vi "Translate XBox Controller Data 2.vi"(2 "Steer Axis":i32, 3 "Drive Axis":dbl) -> (0 "Steer Value Output String":string, 1 "Drive Value Output String":string)   [LabVIEW 2011]
uses:
  <vilib>/express/express arith-compare/Formula/XNode/ExpressFormulaBlockNode.xnode
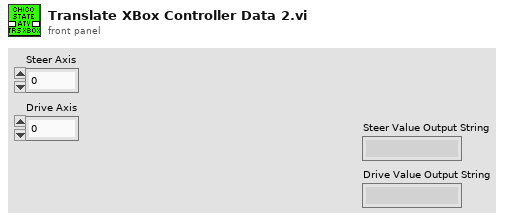
[diagram p1: front panel]
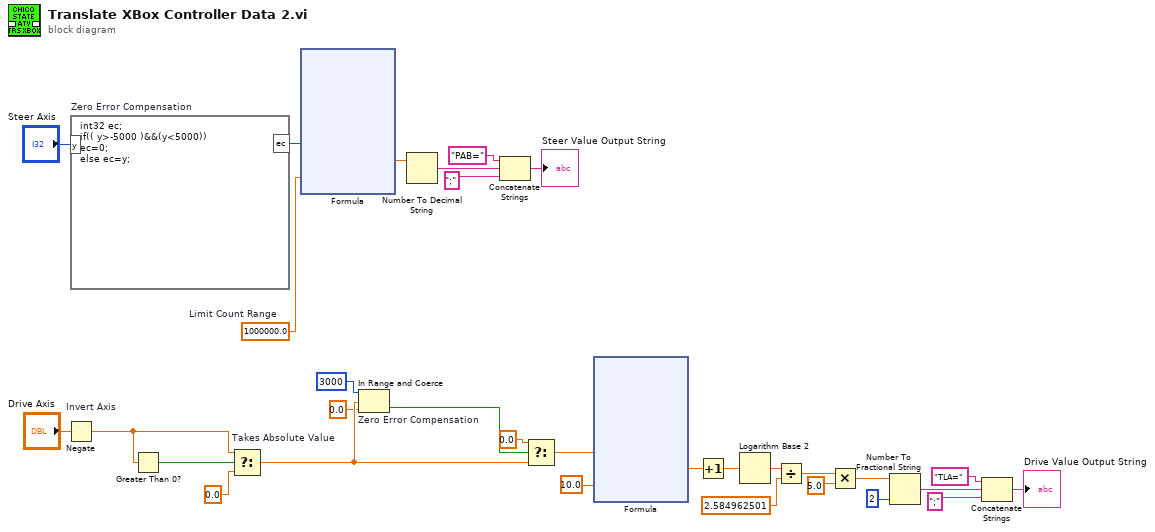
[diagram p0: block diagram]
diagram:
  w18 = 1000000.0  # Limit Count Range
  n1 = Negate "Invert Axis"(x="Drive Axis") -> (-x=w30:dbl)
  n2 = formula code="int32 ec;\nif(( y>-5000 )&&(y<5000))\nec=0;\nelse ec=y;" "Zero Error Compensation"("y"="Steer Axis") -> ("ec"=w21:i32)
  n3 = Greater Than 0?(x=w30) -> (x > 0?=w31:bool)
  n4 = Select "Takes Absolute Value"(t=w30, s=w31, f=0.0) -> (s? t:f=w27:dbl)
  n5 = xnode "Formula"("X1"=w21, "X2"=w18) -> ("Result"=w8:dbl)  [unwired: 1 in, 1 out]
  n6 = In Range and Coerce "Zero Error Compensation"(upper limit=3000, x=w27, lower limit=0.0) -> (In Range?=w28:bool)  [unwired: 1 out]
  n7 = Number To Decimal String(number=w8) -> (decimal integer string=w12:string)  [unwired: 1 in]
  n8 = Concatenate Strings("PAB=" ("string"), w12, ";" ("string")) -> (→"Steer Value Output String":string)
  n9 = Select(t=0.0, s=w28, f=w27) -> (s? t:f=w20:dbl)
  n10 = xnode "Formula"("X1"=w20, "X2"=10.0) -> ("Result"=w7:dbl)  [unwired: 1 in, 1 out]
  n11 = Increment(x=w7) -> (x+1=w6:dbl)
  n12 = Logarithm Base 2(1:w6) -> (0:w5:dbl)
  n13 = Divide(x=w5, y=2.584962501) -> (x/y=w3:dbl)
  n14 = Multiply(x=w3, y=5.0) -> (x*y=w1:dbl)
  n15 = Number To Fractional String(number=w1, precision (6)=i16 2) -> (F-format string=w10:string)  [unwired: 2 in]
  n16 = Concatenate Strings("TLA=" ("string"), w10, ";" ("string")) -> (→"Drive Value Output String":string)
